vi "EEI EXP1.vi"() -> ()   [LabVIEW 2020]
panel:
  in  "X 1":dbl
  in  "X 2":dbl
  out "Slope":dbl
  in  "Y 1":dbl
  in  "Y 2":dbl
  out "Fahrenheit":dbl
  in  "Celcius":dbl
  out "Average":dbl
  in  "Input 2":dbl
  in  "Input 1":dbl
  out "current time":timestamp
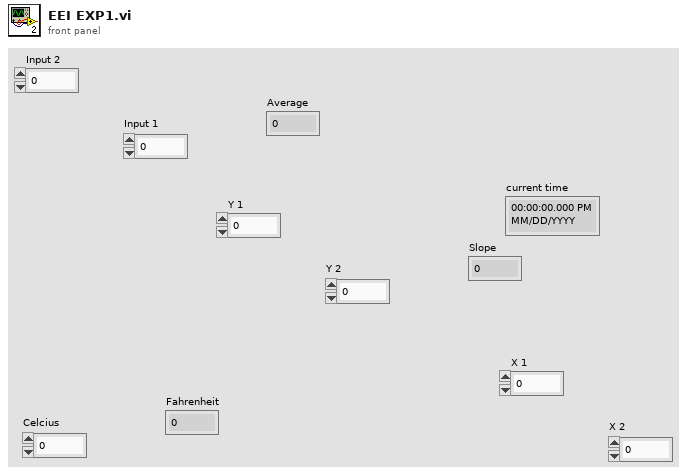
[diagram p1: front panel]
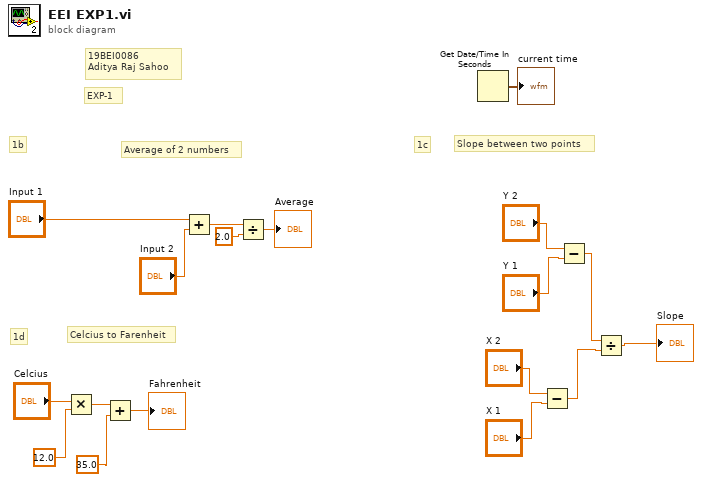
[diagram p0: block diagram]
diagram:
  # "Slope between two points"
  # "Celcius to Farenheit"
  # "Average of 2 numbers"
  # "1d"
  # "1c"
  # "1b"
  # "19BEI0086\nAditya Raj Sahoo"
  # "EXP-1"
  n1 = Multiply(x="Celcius", y=12.0) -> (x*y=w11:dbl)
  n2 = Add(x=w11, y=35.0) -> (x+y=→"Fahrenheit":dbl)
  n3 = Add(x="Input 1", y="Input 2") -> (x+y=w14:dbl)
  n4 = Divide(x=w14, y=2.0) -> (x/y=→"Average":dbl)
  n5 = Get Date/Time In Seconds() -> (seconds since 1Jan1904=→"current time":timestamp)
  n6 = Subtract(x="X 2", y="X 1") -> (x-y=w1:dbl)
  n7 = Subtract(x="Y 2", y="Y 1") -> (x-y=w4:dbl)
  n8 = Divide(x=w4, y=w1) -> (x/y=→"Slope":dbl)
